vi "CLC_CMD_Module.vi"(7 "CMD in":string, 8 "error in":errorcluster, 11 "TCPIPin":T1={"address"="192.168.100.111", "remote port or service name"=5025, "timeout ms (60000)"=10000}) -> (0 "error out":errorcluster, 1 "data out":string, 2 "OK?":bool, 3 "TCPIPout":T1={"address"="192.168.100.111", "remote port or service name"=5025, "timeout ms (60000)"=10000})   [LabVIEW 2023]
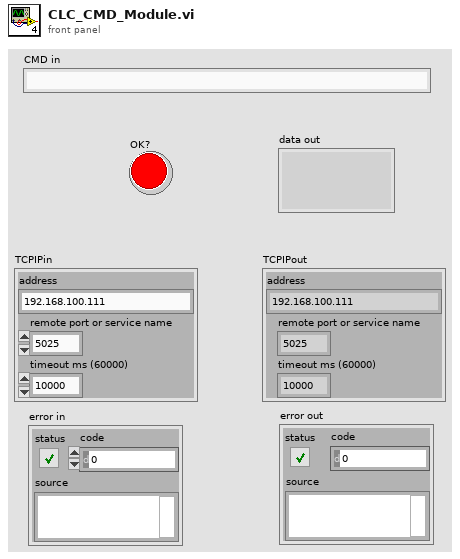
[diagram p1: front panel]
types:
  T1 = cluster{"address":string, "remote port or service name":u16, "timeout ms (60000)":i32}
  T2 = enum16{"Standard", "Buffered", "CRLF", "Immediate"}
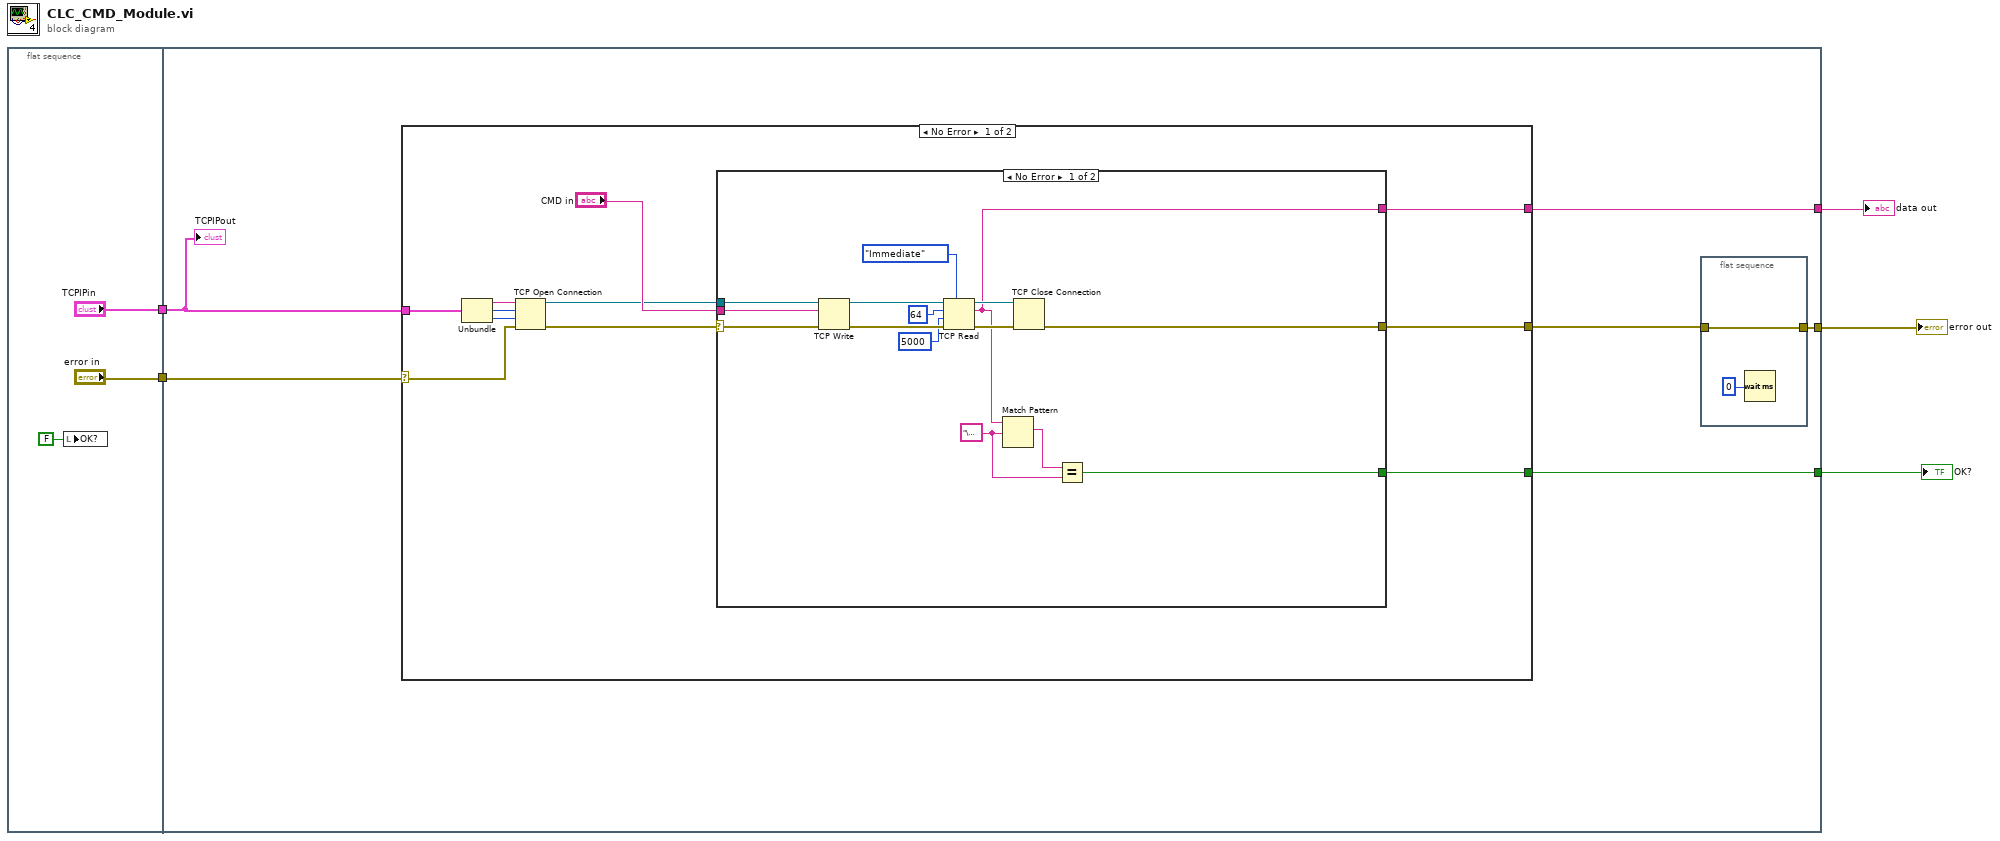
[diagram p0: block diagram]
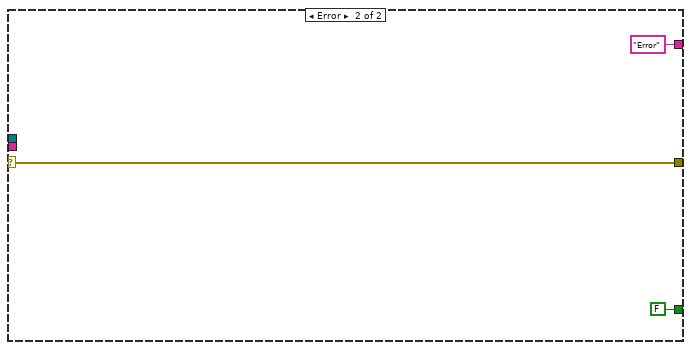
[diagram p2: hidden frame]
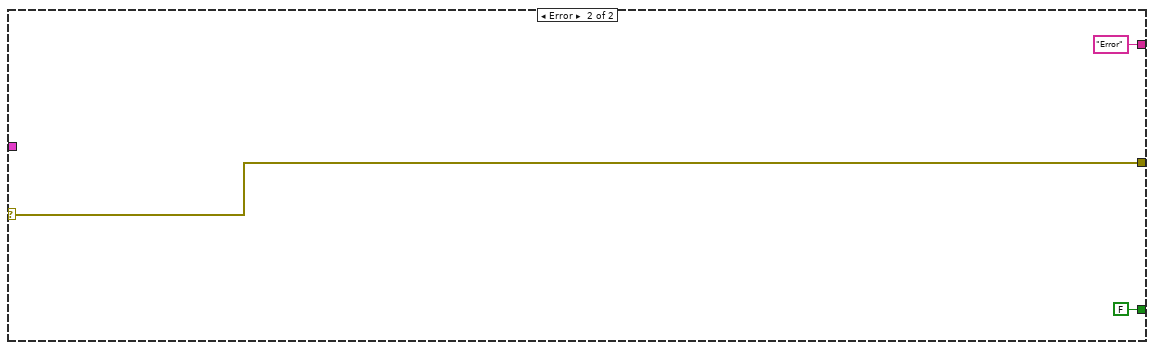
[diagram p3: hidden frame]
diagram:
  n1 = flat-sequence {
    tunnel: ["TCPIPin"] -> w5
    tunnel: ["error in"] -> w4
    tunnel: w5 -> [w14]
    tunnel: w4 -> [w11]
    tunnel: [w13] -> w3
    tunnel: [w12] -> w2
    tunnel: [w10] -> w1
    frame #0 {
      n2 = local write "OK?"(FALSE ("OK?")) -> ()
    }
    frame #1 {
      n3 = case shown="No Error" w11 {
        selector: w11 -> [w17 w46]
        tunnel: w14 -> [w19 _]
        tunnel: [w18 FALSE] -> w12
        tunnel: [w16 "Error" ("data out")] -> w10
        tunnel: [w24 w46] -> w9
        frame No Error {
          n4 = Unbundle(w19) -> ("address"=w21:string, "remote port or service name"=w22:u16, "timeout ms (60000)"=w23:i32)
          n5 = TCP Open Connection(address=w21, remote port or service name=w22, timeout ms (60000)=w23, error in (no error)=w17) -> (connection ID=w20:refnum<k5>, error out=w15:errorcluster)  [unwired: 1 in]
          n6 = case shown="No Error" w15 {
            selector: w15 -> [w26 w43]
            tunnel: "CMD in" -> [w40 _]
            tunnel: [w39 w43] -> w24
            tunnel: w20 -> [w33 _]
            tunnel: [w28 FALSE] -> w18
            tunnel: [w27 "Error" ("data out")] -> w16
            frame No Error {
              w32 = "\u0000" ("string")
              n7 = TCP Write(connection ID=w33, data in=w40, error in (no error)=w26) -> (connection ID out=w35:refnum<k5>, error out=w34:errorcluster)  [unwired: 1 in, 1 out]
              n8 = TCP Read(connection ID=w35, bytes to read=64, error in (no error)=w34, 7:T2."Immediate" ("mode (standard)"), 9:5000 ("timeout ms (25000)")) -> (connection ID out=w36:refnum<k5>, data out=w27:string, error out=w37:errorcluster)
              n9 = Match Pattern(string=w27, regular expression=w32) -> (match substring=w38:string)  [unwired: 1 in, 3 out]
              n10 = TCP Close Connection(connection ID=w36, error in (no error)=w37) -> (error out=w39:errorcluster)  [unwired: 1 in, 1 out]
              n11 = Equal?(x=w38, y=w32) -> (x = y?=w28:bool)
            }
            frame Error {
            }
          }
        }
        frame Error {
        }
      }
      n12 = flat-sequence {
        tunnel: w9 -> [w48]
        tunnel: [w48] -> w13
        frame #0 {
          n13 = Wait (ms)(milliseconds to wait=u32 0) -> ()  [unwired: 1 out]
        }
      }
      "TCPIPout" <- w14
    }
  }
  "error out" <- w3
  "OK?" <- w2
  "data out" <- w1
